vi "Add Copyright.vi"(7 "VI Index":i32, 8 "error in (no error)":errorcluster, 9 "Copyright Delimiter":string, 10 "Copyright Text":string, 11 "Item Data":refnum<class "Item.lvclass">[](array[class])) -> (0 "error out":errorcluster, 3 "Item Data out":refnum<class "Item.lvclass">[](array[class]))   [LabVIEW 2020, in "VI Properties Editor.lvlib"]
doc: "Adds <B>Copyright Text</B> to the VI identified by <B>VI Index</B>. If that value is -1, adds the text to all VIs."
uses:
  VI Properties Editor.lvlib
  Classes/Item/Item.lvclass
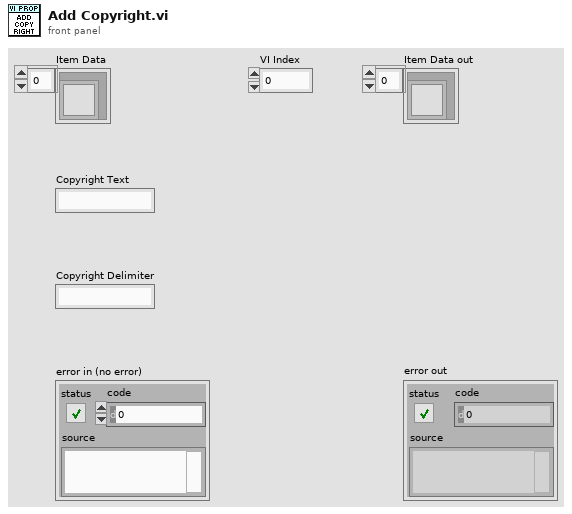
[diagram p1: front panel]
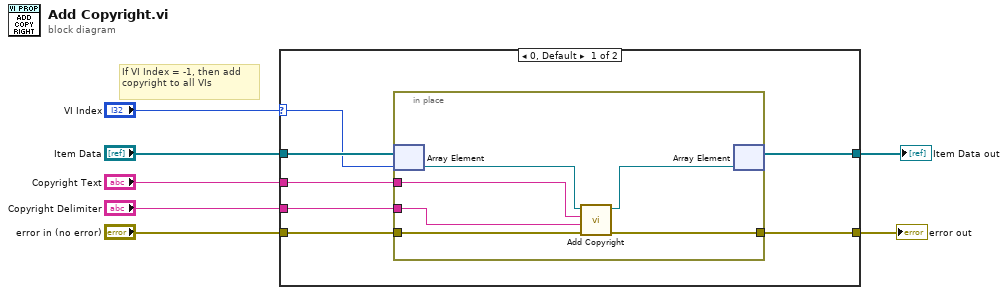
[diagram p0: block diagram]
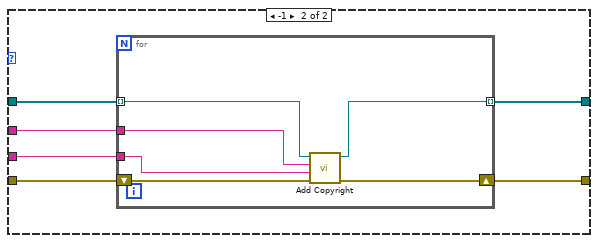
[diagram p2: hidden frame]
diagram:
  # "If VI Index = -1, then add copyright to all VIs"
  n1 = case shown="0, Default" "VI Index" {
    selector: "VI Index" -> [w13 _]
    tunnel: "Item Data" -> [w14 w26]
    tunnel: "Copyright Text" -> [w12 w25]
    tunnel: [w11 w24] -> w3
    tunnel: "error in (no error)" -> [w10 w23]
    tunnel: [w9 w22] -> w2
    tunnel: "Copyright Delimiter" -> [w8 w21]
    frame 0, Default {
      n2 = in-place {
        in-place-border: w12 -> [w17]
        in-place-border: w10 -> [w19]
        in-place-border: [w16] -> w9
        in-place-border: w8 -> [w15]
        n3 = in-place-array #1(w14, w13) -> (w20:refnum<class "Item.lvclass">)
        n4 = call-dynamic "Add Copyright.vi"("error in (no error)"=w19, "Delimiter"=w15, "Copyright"=w17, "Item in"=w20) -> ("error out"=w16:errorcluster, "Item out"=w18:refnum<class "Item.lvclass">)  [unwired: 6 in]
        n5 = in-place-array #1(w18) -> (w11:refnum<class "Item.lvclass">[])  [unwired: 1 out]
      }
    }
    frame -1 {
      n6 = for {
        tunnel: w26 -> [w30] mode=indexing
        tunnel: w25 -> [w29]
        tunnel: [w31] -> w24 mode=indexing
        shift-right: [w28] -> w22
        shift-left: w23 -> [w32]
        tunnel: w21 -> [w27]
        n7 = call-dynamic "Add Copyright.vi"("error in (no error)"=w32, "Delimiter"=w27, "Copyright"=w29, "Item in"=w30) -> ("error out"=w28:errorcluster, "Item out"=w31:refnum<class "Item.lvclass">)  [unwired: 6 in]
      }
    }
  }
  "error out" <- w2
  "Item Data out" <- w3
